vi "CSC_SetCuffLocation.vi"(8 "error in (no error)":errorcluster, 10 "Cuff Location":T1, 11 "C-Alex in":refnum<class "CableSerialChain.lvclass">) -> (0 "error out":errorcluster, 3 "C-Alex out":refnum<class "CableSerialChain.lvclass">)   [LabVIEW 2014]
uses:
  Body/xyzO.ctl
  Body/Bodies.lvclass
  CableSerialChain.lvclass
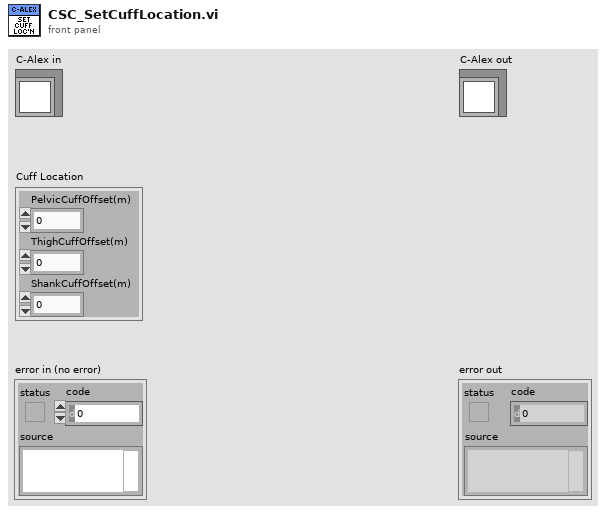
[diagram p1: front panel]
types:
  T1 = cluster{"PelvicCuffOffset(m)":dbl, "ThighCuffOffset(m)":dbl, "ShankCuffOffset(m)":dbl}
  T2 = typedef "Bodies.lvclass/xyzO.ctl" = enum16{"X", "Y", "Z", "O"}
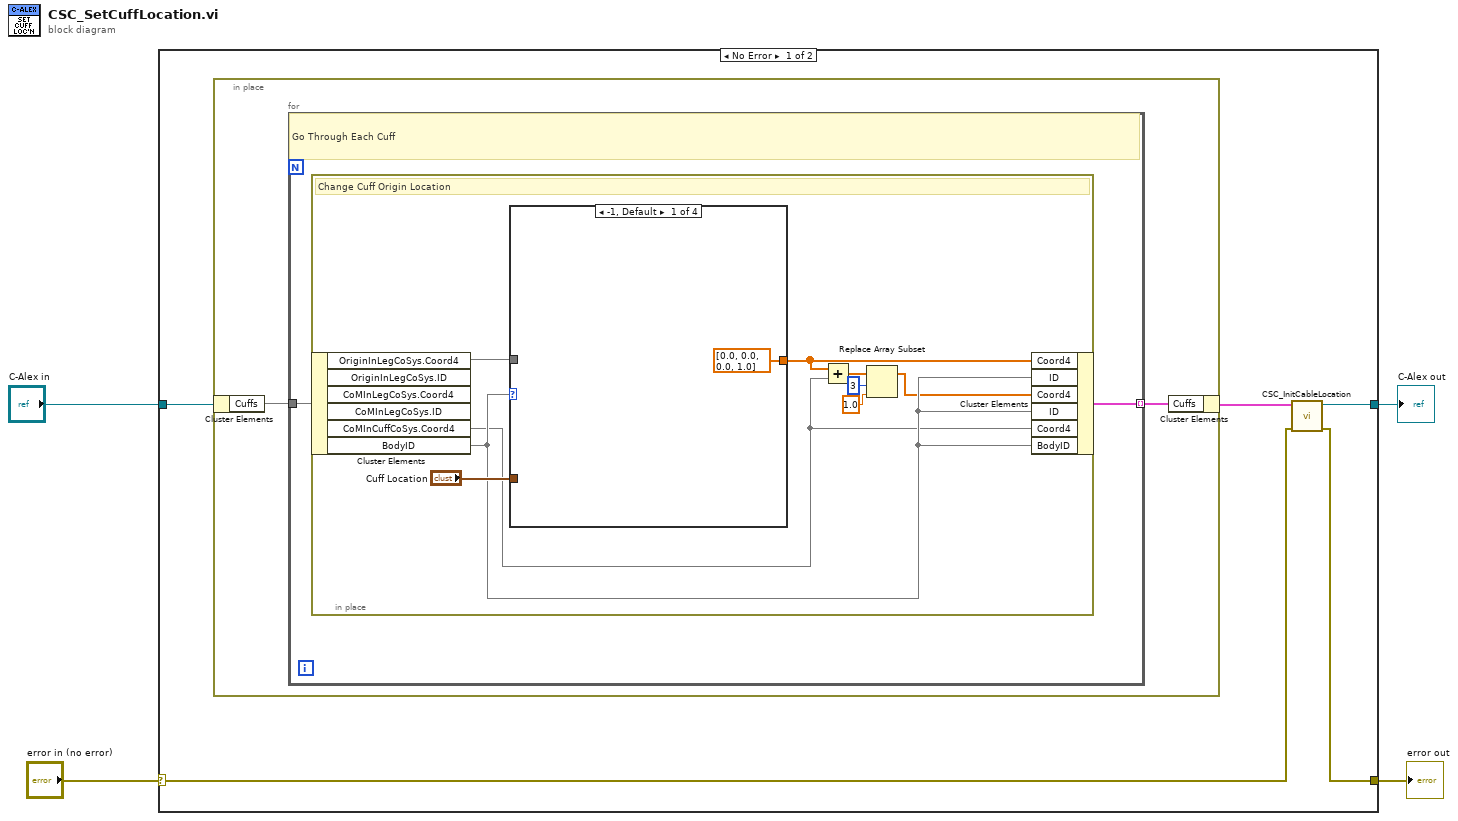
[diagram p0: block diagram]
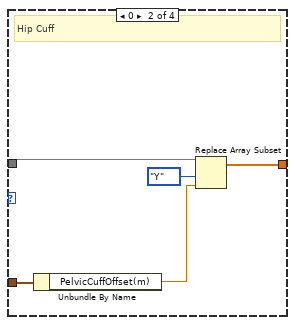
[diagram p2: hidden frame]
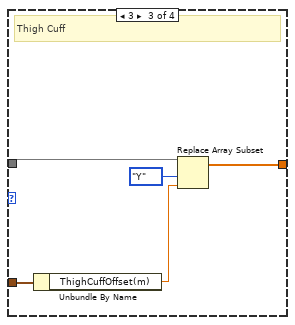
[diagram p3: hidden frame]
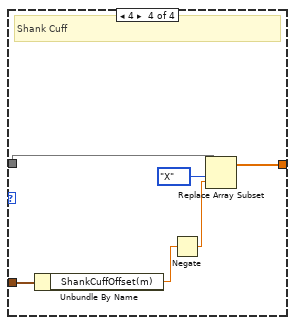
[diagram p4: hidden frame]
diagram:
  n1 = case shown="No Error" "error in (no error)" {
    selector: "error in (no error)" -> [w6 w41]
    tunnel: [w5 w41] -> w3
    tunnel: [w8 w40] -> w1
    tunnel: "C-Alex in" -> [w9 w40]
    frame No Error {
      n2 = in-place {
        n3 = in-place-cluster #1(w9) -> ("Cuffs"=w11)
        n4 = for {
          tunnel: w11 -> [w13]
          tunnel: [w12] -> w10 mode=indexing
          # "Go Through Each Cuff"
          n5 = in-place {
            # "Change Cuff Origin Location"
            n6 = in-place-cluster #2(w13) -> ("OriginInLegCoSys.Coord4"=w21, "CoMInCuffCoSys.Coord4"=w18, "BodyID"=w20)  [unwired: 3 out]
            n7 = case shown="-1, Default" w20 {
              tunnel: "Cuff Location" -> [_ w28 w33 w39]
              tunnel: w21 -> [_ w27 w32 w38]
              tunnel: [dbl[] [0.0, 0.0, 0.0, 1.0] ("Coord4") w24 w29 w35] -> w19
              frame -1, Default {
              }
              frame 0 {
                # "Hip Cuff"
                n8 = Unbundle By Name(w28) -> ("PelvicCuffOffset(m)"=w26:dbl)
                n9 = Replace Array Subset(array=w27, new element=w26, index=xyzO."Y" ("XYZ")) -> (w24:dbl[])
              }
              frame 3 {
                # "Thigh Cuff"
                n10 = Unbundle By Name(w33) -> ("ThighCuffOffset(m)"=w31:dbl)
                n11 = Replace Array Subset(array=w32, new element=w31, index=xyzO."Y" ("XYZ")) -> (w29:dbl[])
              }
              frame 4 {
                # "Shank Cuff"
                n12 = Unbundle By Name(w39) -> ("ShankCuffOffset(m)"=w37:dbl)
                n13 = Negate(x=w37) -> (-x=w34:dbl)
                n14 = Replace Array Subset(array=w38, new element=w34, index=xyzO."X" ("XYZ")) -> (w35:dbl[])
              }
            }
            n15 = Add(x=w19, y=w18) -> (x+y=w17:dbl[])
            n16 = Replace Array Subset(array=w17, new element=1.0 ("new element/subarray"), index=3) -> (w16:dbl[])
            n17 = in-place-cluster #2("Coord4"=w19, "ID"=w20, "Coord4"=w16, "ID"=w20, "Coord4"=w18, "BodyID"=w20) -> (w12:cluster{})
          }
        }
        n18 = in-place-cluster #1("Cuffs"=w10) -> (w7:cluster{})
      }
      n19 = call "CSC_InitCableLocation.vi"("error in (no error)"=w6, "C-Alex in"=w7) -> ("error out"=w5:errorcluster, "C-Alex out"=w8:refnum<class "CableSerialChain.lvclass">)  [unwired: 8 in]
    }
    frame Error {
    }
  }
  "error out" <- w3
  "C-Alex out" <- w1
